vi "pressure system controller v14 motor.vi"() -> ()   [LabVIEW 2009]
uses:
  <vilib>/DAQmx/create/channels.llb/DAQmx Create Channel (DO-Digital Output).vi
  <vilib>/Instr/_visa.llb/VISA Configure Serial Port (Instr).vi
  <vilib>/DAQmx/write.llb/DAQmx Write (Digital 1D Bool 1Chan 1Samp).vi
  <instrlib>/Keithley 24XX/Public/Data/Read (Single Point).vi
  <vilib>/express/express signal manip/GetorSetDDTAttributes/Set DDT Attributes/Set DDT Properties.xnode
  <vilib>/express/express shared/transition.llb/Waveform Array To Dynamic.vi
  <vilib>/express/express signal manip/GetorSetDDTAttributes/Set DDT Attributes/SetT0.vi
  <vilib>/express/express shared/transition.llb/Dynamic To Waveform Array.vi
  <instrlib>/Keithley 24XX/Keithley 24XX.lvlib
  <instrlib>/Agilent E4980/Agilent E4980.lvlib
panel:
  in  "Pressure (mmHg)":i32
  out "error out":errorcluster
  in  "motor GO!":bool
  in  "stop":bool
  in  "MUX4: Keithley (-)":T1(radio)
  in  "MUX3: Keithley (+)":T1(radio)
  in  "MUX2: LCR (-)":T1(radio)
  in  "MUX1: LCR (+)":T1(radio)
  in  "Write to file":bool=TRUE caption="Enable"
  in  "Turn on (MAKE SURE TURN OFF)":bool=TRUE
  out "Impedance":dbl format="%^#_4e"
  out "Phase (deg)":dbl
  in  "Function (0: Cp-D)":u16(ring)=17 items=["Cp-D", "Cp-Q", "Cp-G", "Cp-Rp", "Cs-D", "Cs-Q", "Cs-Rs", "Lp-D", "Lp-Q", "Lp-G", "Lp-Rp", "Lp-Rdc", "Ls-D", "Ls-Q", "Ls-Rs", "Ls-Rdc", "R-X", "Z-thd", "Z-thr", "G-B", "Y-thd", "Y-thr", "Vdc-Idc"]
  in  "Signal Level (1.0 V)":dbl=1.0
  in  "Averaging Factor (1)":i32=1
  in  "Measurement Time (1: Medium)":u16(ring) items=["Short", "Medium", "Long"]
  in  "Signal Frequency":dbl=10000.0
  out "Resistance (Mohm)":dbl
  out "Current (uA)":sgl
  out "Voltage":sgl
  in  "Loop sample rate (samples per second)":dbl=5.0
  in  "Current duration (s)":dbl=2.0
  out "Time Counter":i32
  in  "Keithley Output (uA)":dbl=1.0
  in  "Compliance (V)":dbl=21.0
  in  "Inject Current":bool
  # "Switch"
  # "Keithley Settings"
  # "LCR Settings"
  # "1KHz for water"
  # "10KHz for PBS"
  # "1 uA minimum"
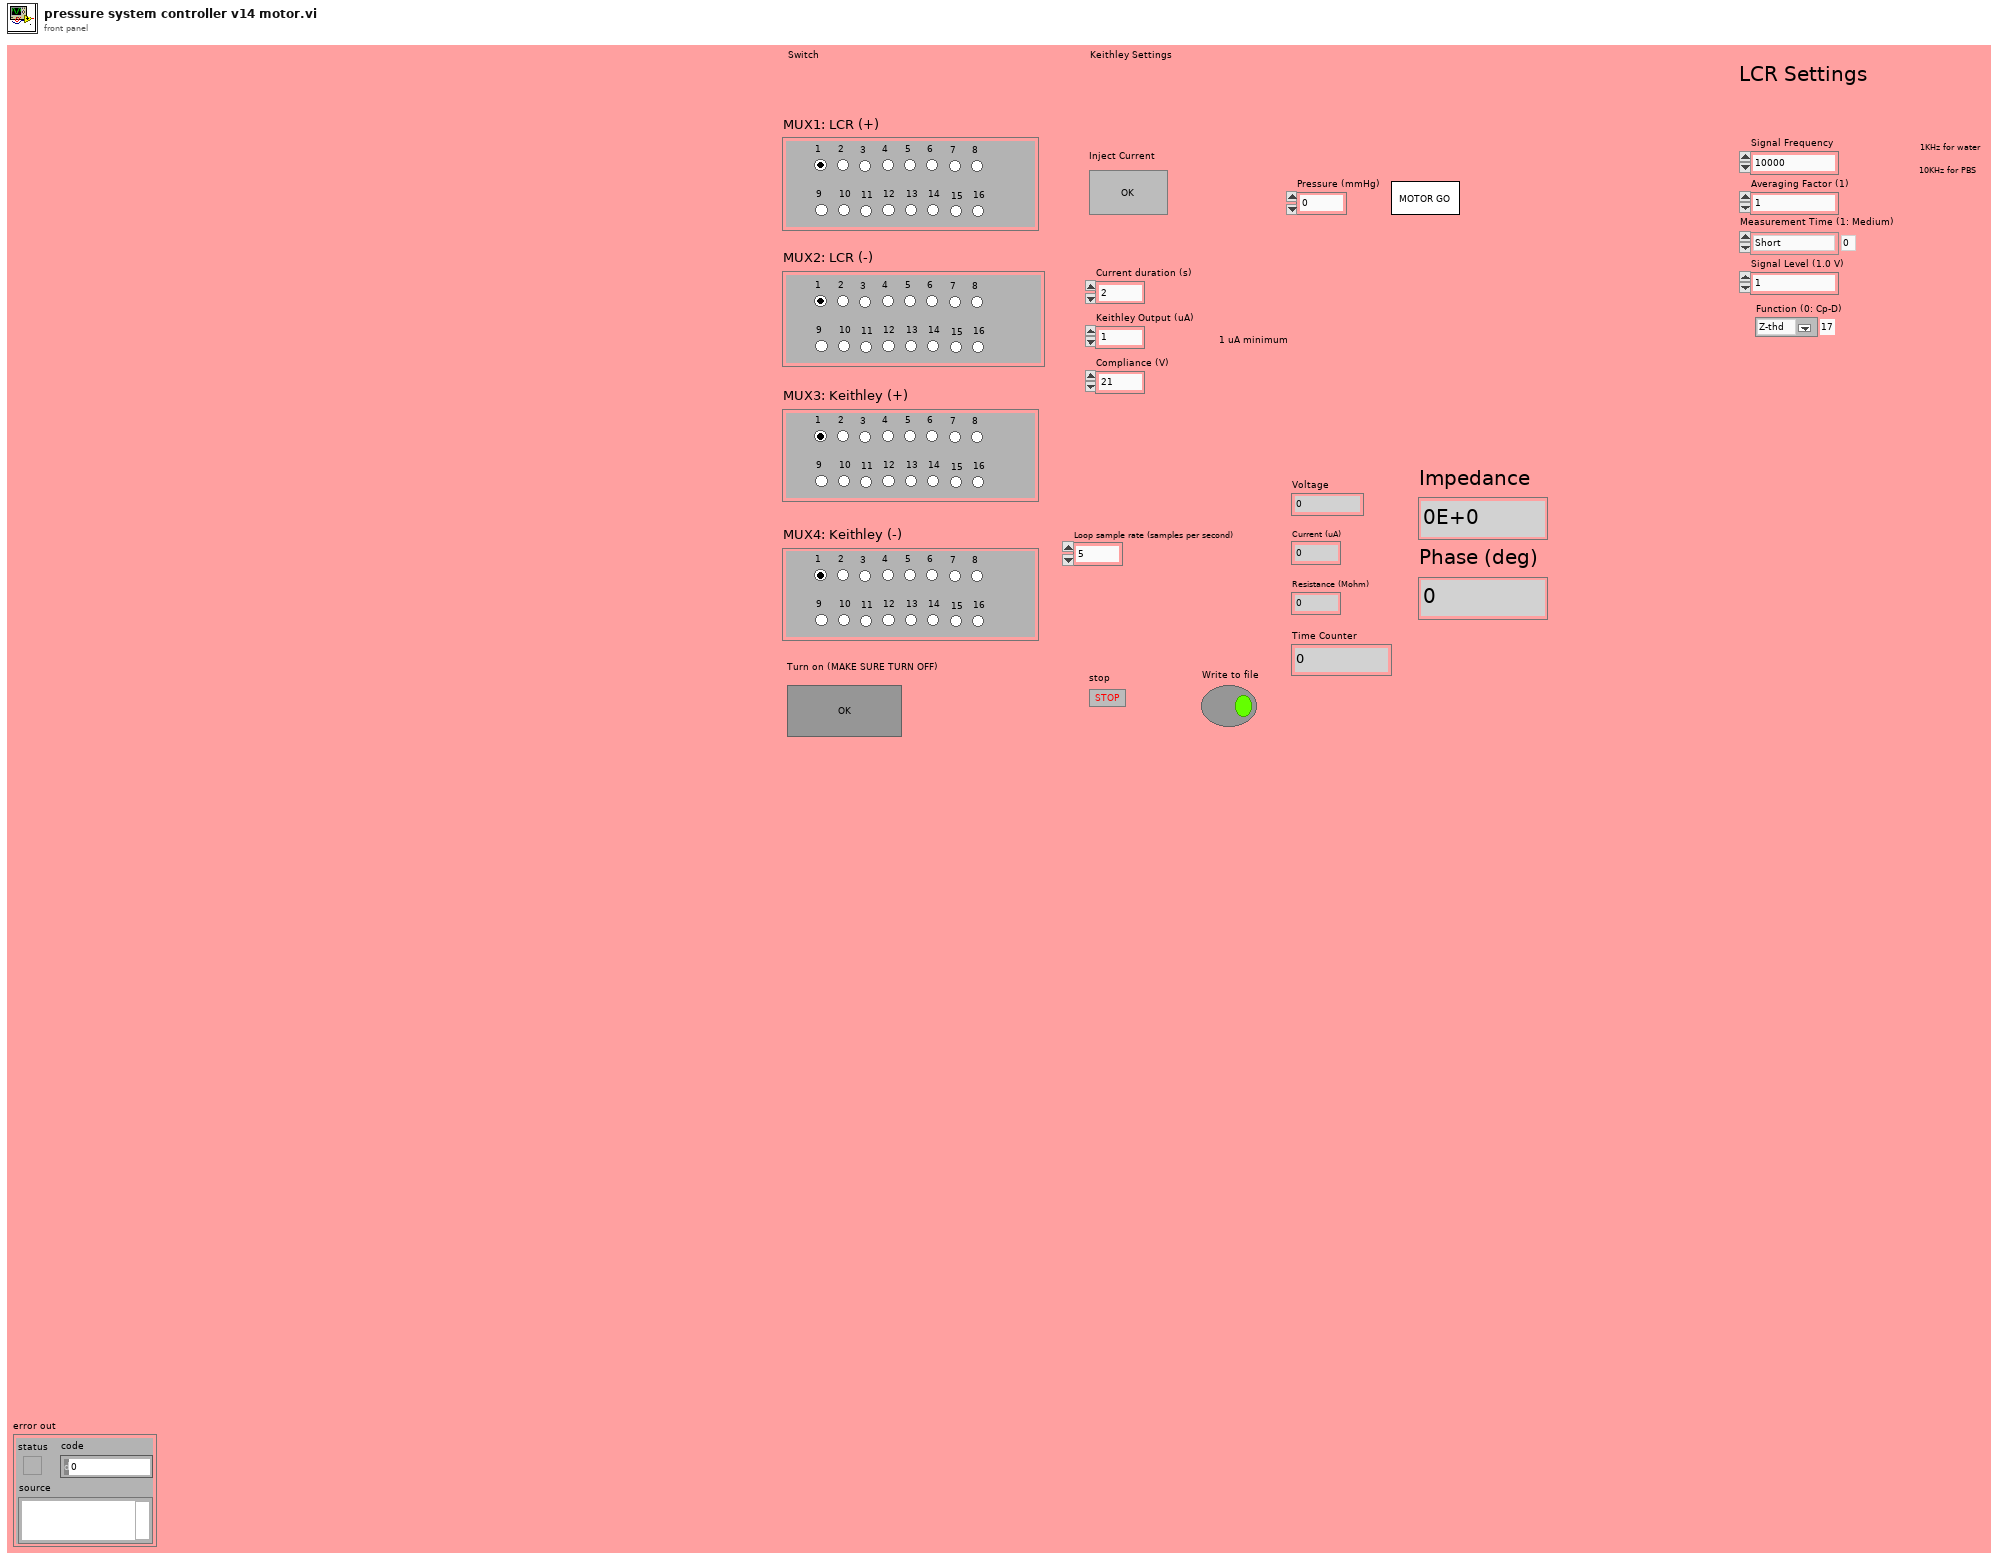
[diagram p1: front panel]
types:
  T1 = enum32{"1", "2", "3", "4", "5", "6", "7", "8", "9", "10", "11", "12", "13", "14", "15", "16"}
  T2 = cluster{"Primary Parameter":dbl, "Secondary Parameter":dbl}
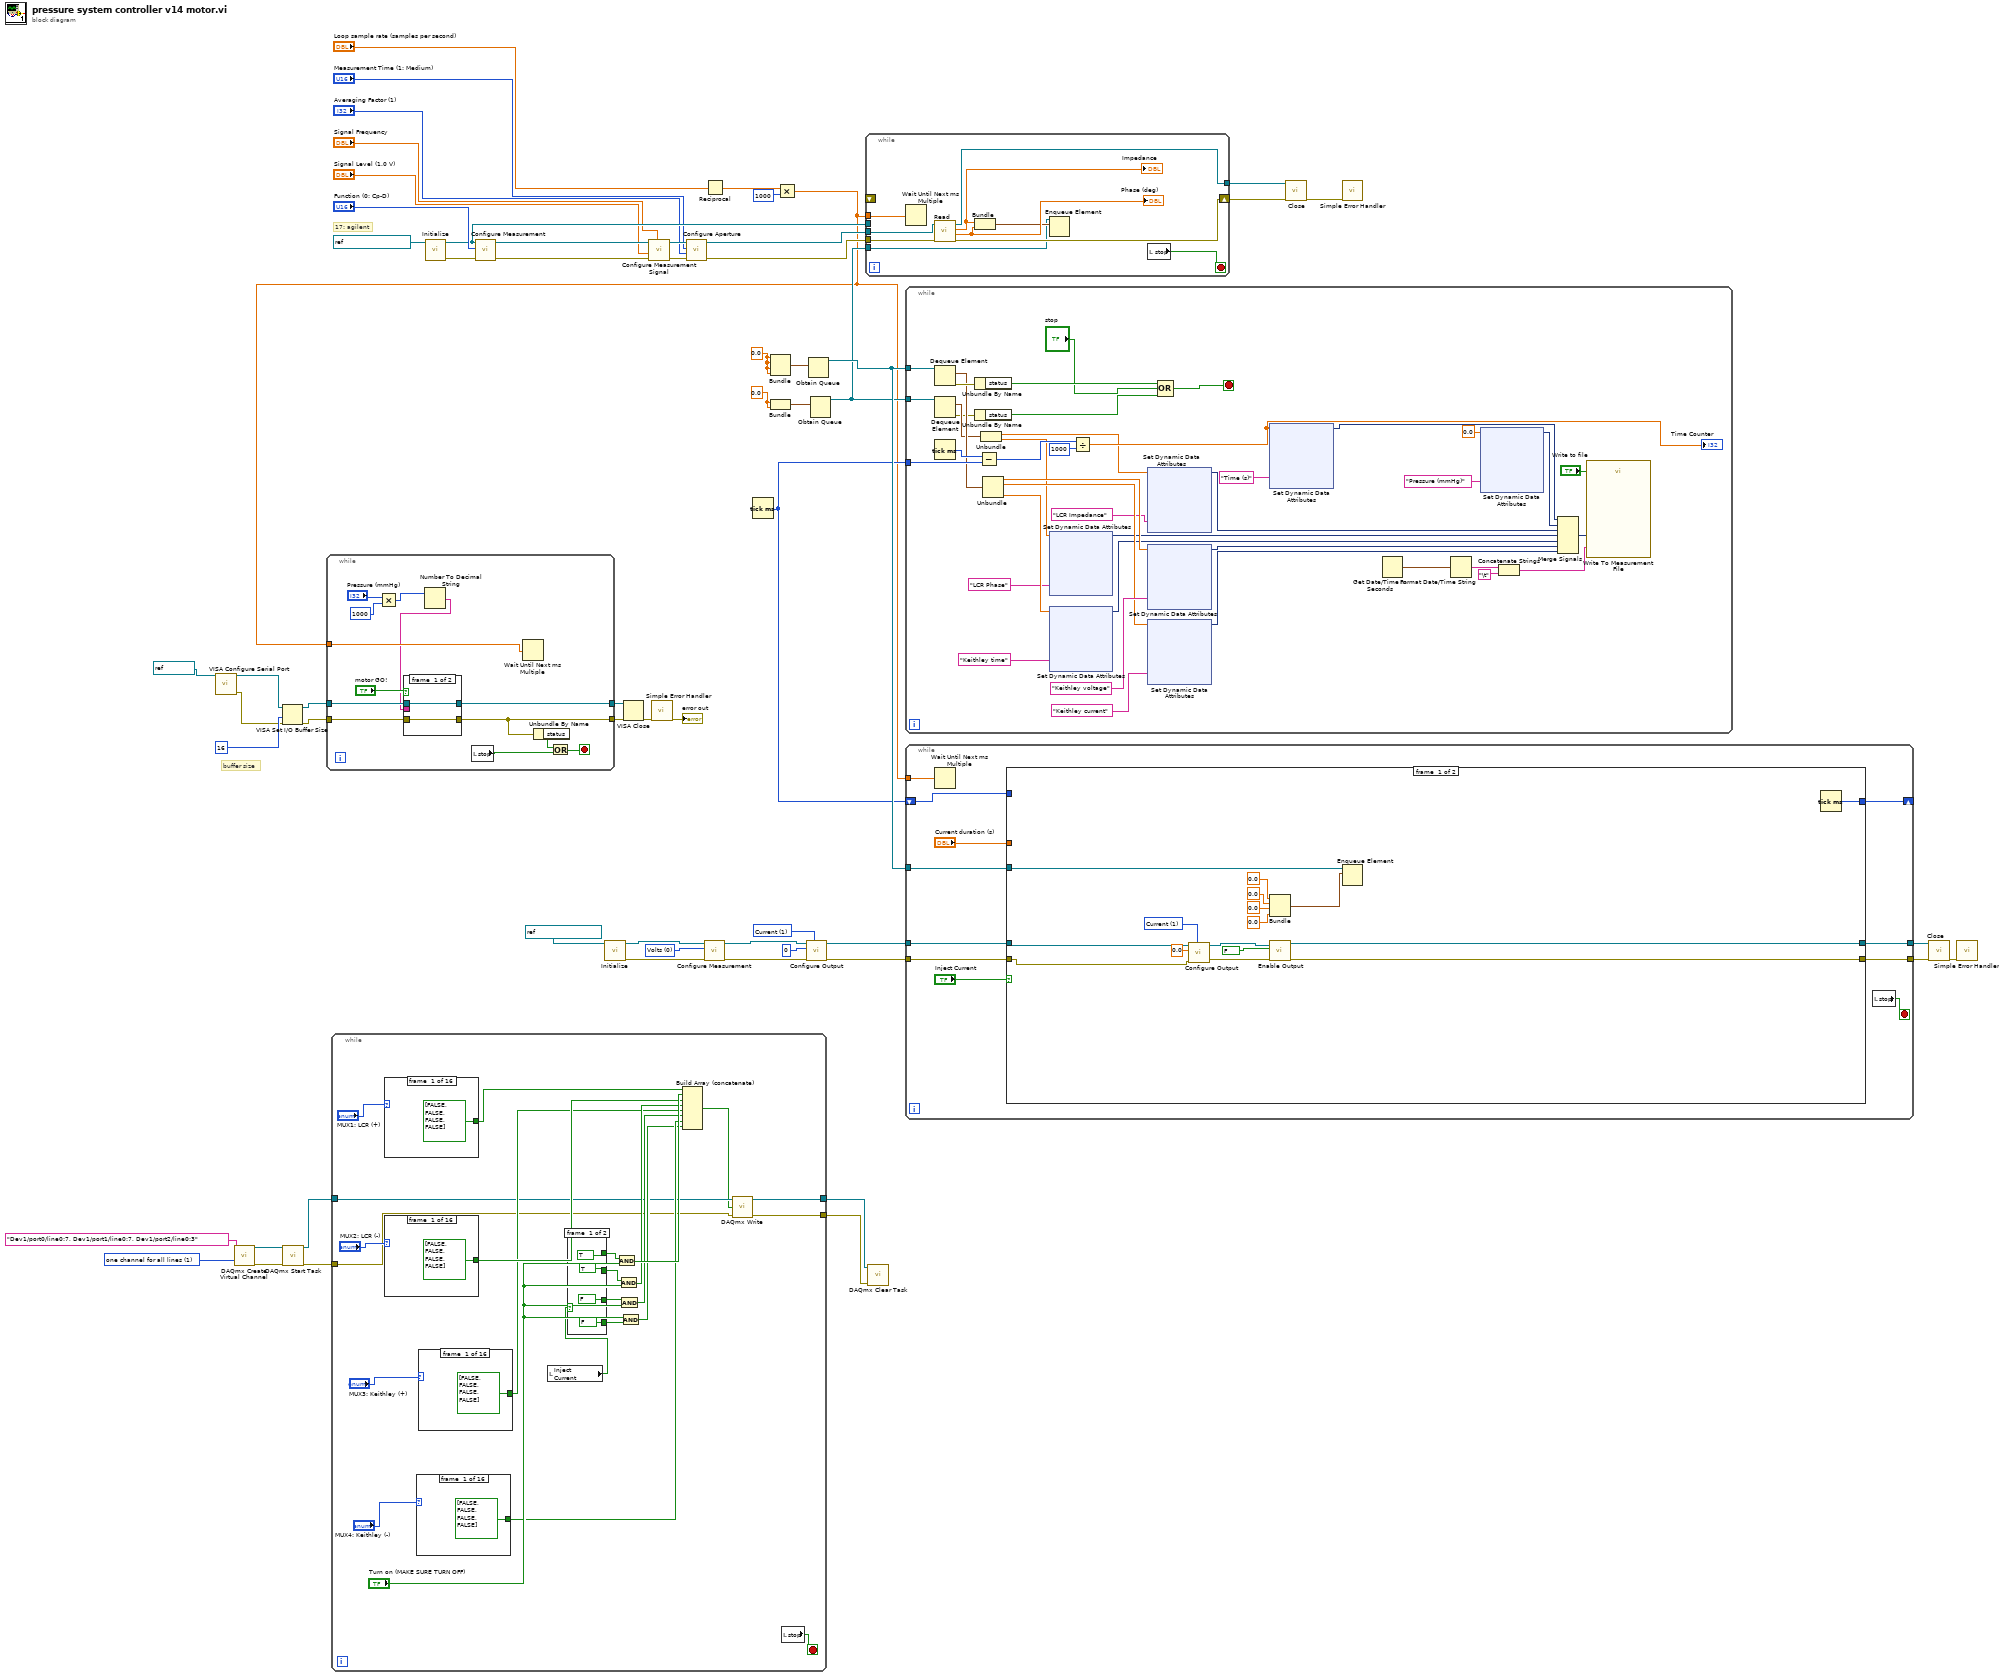
[diagram p0: block diagram]
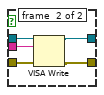
[diagram p2: hidden frame]
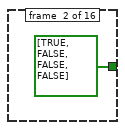
[diagram p3: hidden frame]
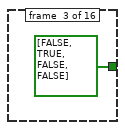
[diagram p4: hidden frame]
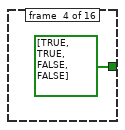
[diagram p5: hidden frame]
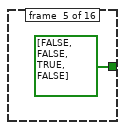
[diagram p6: hidden frame]
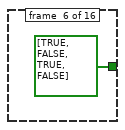
[diagram p7: hidden frame]
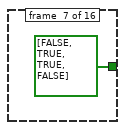
[diagram p8: hidden frame]
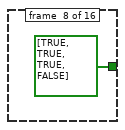
[diagram p9: hidden frame]
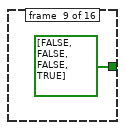
[diagram p10: hidden frame]
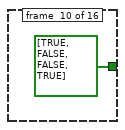
[diagram p11: hidden frame]
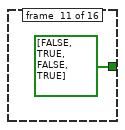
[diagram p12: hidden frame]
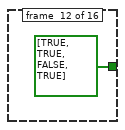
[diagram p13: hidden frame]
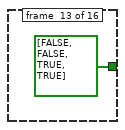
[diagram p14: hidden frame]
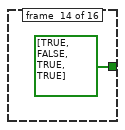
[diagram p15: hidden frame]
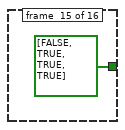
[diagram p16: hidden frame]
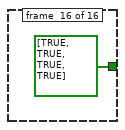
[diagram p17: hidden frame]
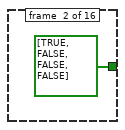
[diagram p18: hidden frame]
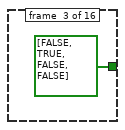
[diagram p19: hidden frame]
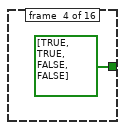
[diagram p20: hidden frame]
diagram:
  w20 = 1 items=["one channel for each line", "one channel for all lines"] ("line grouping")
  w53 = u16 1 items=["Voltage", "Current"] ("Source Mode  (0: Voltage)")
  w59 = u16 0 items=["Volts", "Current", "Resistance"] ("Keithley Measure")
  w39 = sgl 0.0 ("y")
  w47 = sgl 0.0 ("y")
  # "buffer size"
  # "17: agilent"
  n1 = call-poly "VISA Configure Serial Port"("VISA resource name"=refnum<visa-resource-name> "COM3") -> ("VISA resource name out"=w4:refnum<visa-resource-name>, "error out"=w3:errorcluster)  [unwired: 13 in]
  n2 = call-poly <vilib>:"DAQmx Create Virtual Channel.vi"("lines"=tag "Dev1/port0/line0:7, Dev1/port1/line0:7, Dev1/port2/line0:3", "line grouping"=w20) -> ("task out"=w18:refnum<k21>, "error out"=w19:errorcluster)  [unwired: 12 in]
  n3 = VISA Set I/O Buffer Size(VISA resource name=w4, size (4096)=u32 16 ("buffer size"), error in (no error)=w3) -> (VISA resource name out=w5:refnum<visa-resource-name>, error out=w6:errorcluster)  [unwired: 1 in]
  n4 = call <vilib>:"DAQmx Start Task.vi"("task/channels in"=w18, "error in"=w19) -> ("task out"=w16:refnum<k21>, "error out"=w14:errorcluster)  [unwired: 12 in]
  n5 = while {
    tunnel: w16 -> [w65]
    tunnel: [w64] -> w15
    tunnel: w14 -> [w63]
    tunnel: [w62] -> w13
    stop <- w82 stop-if-true
    n6 = case shown="\"1\", Default" "MUX1: LCR (+)" {
      tunnel: [bool[] [FALSE, FALSE, FALSE, FALSE] bool[] [TRUE, FALSE, FALSE, FALSE] bool[] [FALSE, TRUE, FALSE, FALSE] bool[] [TRUE, TRUE, FALSE, FALSE] bool[] [FALSE, FALSE, TRUE, FALSE] bool[] [TRUE, FALSE, TRUE, FALSE] bool[] [FALSE, TRUE, TRUE, FALSE] bool[] [TRUE, TRUE, TRUE, FALSE] bool[] [FALSE, FALSE, FALSE, TRUE] bool[] [TRUE, FALSE, FALSE, TRUE] bool[] [FALSE, TRUE, FALSE, TRUE] bool[] [TRUE, TRUE, FALSE, TRUE] bool[] [FALSE, FALSE, TRUE, TRUE] bool[] [TRUE, FALSE, TRUE, TRUE] bool[] [FALSE, TRUE, TRUE, TRUE] bool[] [TRUE, TRUE, TRUE, TRUE]] -> w73
      frame #0 {
      }
      frame #1 {
      }
      frame #2 {
      }
      frame #3 {
      }
      frame #4 {
      }
      frame #5 {
      }
      frame #6 {
      }
      frame #7 {
      }
      frame #8 {
      }
      frame #9 {
      }
      frame #10 {
      }
      frame #11 {
      }
      frame #12 {
      }
      frame #13 {
      }
      frame #14 {
      }
      frame #15 {
      }
    }
    n7 = case shown="\"1\", Default" "MUX2: LCR (-)" {
      tunnel: [bool[] [FALSE, FALSE, FALSE, FALSE] bool[] [TRUE, FALSE, FALSE, FALSE] bool[] [FALSE, TRUE, FALSE, FALSE] bool[] [TRUE, TRUE, FALSE, FALSE] bool[] [FALSE, FALSE, TRUE, FALSE] bool[] [TRUE, FALSE, TRUE, FALSE] bool[] [FALSE, TRUE, TRUE, FALSE] bool[] [TRUE, TRUE, TRUE, FALSE] bool[] [FALSE, FALSE, FALSE, TRUE] bool[] [TRUE, FALSE, FALSE, TRUE] bool[] [FALSE, TRUE, FALSE, TRUE] bool[] [TRUE, TRUE, FALSE, TRUE] bool[] [FALSE, FALSE, TRUE, TRUE] bool[] [TRUE, FALSE, TRUE, TRUE] bool[] [FALSE, TRUE, TRUE, TRUE] bool[] [TRUE, TRUE, TRUE, TRUE]] -> w71
      frame #0 {
      }
      frame #1 {
      }
      frame #2 {
      }
      frame #3 {
      }
      frame #4 {
      }
      frame #5 {
      }
      frame #6 {
      }
      frame #7 {
      }
      frame #8 {
      }
      frame #9 {
      }
      frame #10 {
      }
      frame #11 {
      }
      frame #12 {
      }
      frame #13 {
      }
      frame #14 {
      }
      frame #15 {
      }
    }
    n8 = case shown="\"2\"" "MUX4: Keithley (-)" {
      tunnel: [bool[] [FALSE, FALSE, FALSE, FALSE] bool[] [TRUE, FALSE, FALSE, FALSE] bool[] [FALSE, TRUE, FALSE, FALSE] bool[] [TRUE, TRUE, FALSE, FALSE] bool[] [FALSE, FALSE, TRUE, FALSE] bool[] [TRUE, FALSE, TRUE, FALSE] bool[] [FALSE, TRUE, TRUE, FALSE] bool[] [TRUE, TRUE, TRUE, FALSE] bool[] [FALSE, FALSE, FALSE, TRUE] bool[] [TRUE, FALSE, FALSE, TRUE] bool[] [FALSE, TRUE, FALSE, TRUE] bool[] [TRUE, TRUE, FALSE, TRUE] bool[] [FALSE, FALSE, TRUE, TRUE] bool[] [TRUE, FALSE, TRUE, TRUE] bool[] [FALSE, TRUE, TRUE, TRUE] bool[] [TRUE, TRUE, TRUE, TRUE]] -> w67
      frame #0 {
      }
      frame #1 {
      }
      frame #2 {
      }
      frame #3 {
      }
      frame #4 {
      }
      frame #5 {
      }
      frame #6 {
      }
      frame #7 {
      }
      frame #8 {
      }
      frame #9 {
      }
      frame #10 {
      }
      frame #11 {
      }
      frame #12 {
      }
      frame #13 {
      }
      frame #14 {
      }
      frame #15 {
      }
    }
    n9 = case shown="\"1\", Default" "MUX3: Keithley (+)" {
      tunnel: [bool[] [FALSE, FALSE, FALSE, FALSE] bool[] [TRUE, FALSE, FALSE, FALSE] bool[] [FALSE, TRUE, FALSE, FALSE] bool[] [TRUE, TRUE, FALSE, FALSE] bool[] [FALSE, FALSE, TRUE, FALSE] bool[] [TRUE, FALSE, TRUE, FALSE] bool[] [FALSE, TRUE, TRUE, FALSE] bool[] [TRUE, TRUE, TRUE, FALSE] bool[] [FALSE, FALSE, FALSE, TRUE] bool[] [TRUE, FALSE, FALSE, TRUE] bool[] [FALSE, TRUE, FALSE, TRUE] bool[] [TRUE, TRUE, FALSE, TRUE] bool[] [FALSE, FALSE, TRUE, TRUE] bool[] [TRUE, FALSE, TRUE, TRUE] bool[] [FALSE, TRUE, TRUE, TRUE] bool[] [TRUE, TRUE, TRUE, TRUE]] -> w69
      frame #0 {
      }
      frame #1 {
      }
      frame #2 {
      }
      frame #3 {
      }
      frame #4 {
      }
      frame #5 {
      }
      frame #6 {
      }
      frame #7 {
      }
      frame #8 {
      }
      frame #9 {
      }
      frame #10 {
      }
      frame #11 {
      }
      frame #12 {
      }
      frame #13 {
      }
      frame #14 {
      }
      frame #15 {
      }
    }
    n10 = local read "Inject Current"() -> (w60:bool)
    n11 = case shown="False" w60 {
      tunnel: [TRUE FALSE] -> w77
      tunnel: [TRUE FALSE] -> w76
      tunnel: [FALSE TRUE] -> w75
      tunnel: [FALSE TRUE] -> w74
      frame #0 {
      }
      frame #1 {
      }
    }
    n12 = And(x=w77, y="Turn on (MAKE SURE TURN OFF)") -> (x .and. y?=w72:bool)
    n13 = And(x=w76, y="Turn on (MAKE SURE TURN OFF)") -> (x .and. y?=w70:bool)
    n14 = And(x=w75, y="Turn on (MAKE SURE TURN OFF)") -> (x .and. y?=w68:bool)
    n15 = And(x="Turn on (MAKE SURE TURN OFF)", y=w74) -> (x .and. y?=w66:bool)
    n16 = Build Array (concatenate)(w73, w72, w71, w70, w69, w68, w67, w66) -> (w61:bool[])
    n17 = call-poly <vilib>:"DAQmx Write.vi"("task/channels in"=w65, "data"=w61, "error in"=w63) -> ("task out"=w64:refnum<k21>, "error out"=w62:errorcluster)  [unwired: 10 in, 1 out]
    n18 = local read "stop"() -> (w82:bool)
  }
  n19 = call <instrlib>:"Initialize.vi"("VISA resource name"=refnum<visa-resource-name> "GPIB0::17::INSTR") -> ("error out"=w33:errorcluster, "VISA resource name out"=w32:refnum<visa-resource-name>)  [unwired: 9 in]
  n20 = call <instrlib>:"Configure Measurement.vi"("error in (no error)"=w33, "Function (0: Cp-D)"="Function (0: Cp-D)", "VISA resource name"=w32) -> ("error out"=w31:errorcluster, "VISA resource name out"=w30:refnum<visa-resource-name>)  [unwired: 7 in]
  n21 = call <instrlib>:"Initialize.vi"("VISA resource name"=refnum<visa-resource-name> "GPIB0::24::INSTR") -> ("error out"=w57:errorcluster, "VISA resource name out"=w58:refnum<visa-resource-name>)  [unwired: 9 in]
  n22 = call <instrlib>:"Configure Measurement Signal.vi"("Signal Frequency (1000 Hz)"="Signal Frequency", "error in (no error)"=w31, "Signal Level (1.0 V)"="Signal Level (1.0 V)", "VISA resource name"=w30) -> ("error out"=w27:errorcluster, "VISA resource name out"=w26:refnum<visa-resource-name>)  [unwired: 6 in]
  n23 = call <instrlib>:"Configure Aperture.vi"("error in (no error)"=w27, "Averaging Factor (1)"="Averaging Factor (1)", "Measurement Time (1: Medium)"="Measurement Time (1: Medium)", "VISA resource name"=w26) -> ("error out"=w23:errorcluster, "VISA resource name out"=w22:refnum<visa-resource-name>)  [unwired: 6 in]
  n24 = call <instrlib>:"Configure Measurement.vi"("error in (no error)"=w57, "Function (0: Volts)"=w59, "VISA resource name"=w58) -> ("error out"=w55:errorcluster, "VISA resource name out"=w56:refnum<visa-resource-name>)  [unwired: 7 in]
  n25 = Reciprocal(x="Loop sample rate (samples per second)") -> (1/x=w44:dbl)
  n26 = Tick Count (ms)() -> (millisecond timer value=w12:u32)
  n27 = Bundle("y"=w47, "y"=w47, "y"=w47, "y"=w47) -> (w46:cluster{"y":sgl, "y":sgl, "y":sgl, "y":sgl})  [unwired: 1 in]
  n28 = Bundle("y"=w39, "y"=w39) -> (w38:cluster{"y":sgl, "y":sgl})  [unwired: 1 in]
  n29 = Multiply(x=w44, y=1000) -> (x*y=w2:dbl)
  n30 = while {
    tunnel: w5 -> [w166]
    tunnel: w6 -> [w165]
    tunnel: [w163] -> w11
    tunnel: [w162] -> w10
    tunnel: w2 -> [w161]
    stop <- w167 stop-if-true
    n31 = Multiply(x="Pressure (mmHg)", y=i16 1000) -> (x*y=w157:i32)
    n32 = Number To Decimal String(number=w157) -> (decimal integer string=w159:string)  [unwired: 1 in]
    n33 = case shown="True" "motor GO!" {
      tunnel: w166 -> [w170 w175]
      tunnel: w165 -> [w169 w174]
      tunnel: [w170 w173] -> w163
      tunnel: [w169 w172] -> w162
      tunnel: w159 -> [_ w171]
      frame #0 {
      }
      frame #1 {
        n34 = VISA Write(VISA resource name=w175, write buffer=w171, error in (no error)=w174) -> (VISA resource name out=w173:refnum<visa-resource-name>, error out=w172:errorcluster)  [unwired: 1 out]
      }
    }
    n35 = local read "stop"() -> (w160:bool)
    n36 = Wait Until Next ms Multiple(millisecond multiple=w161) -> ()  [unwired: 1 out]
    n37 = Unbundle By Name(w162) -> ("status"=w168:bool)
    n38 = Or(x=w168, y=w160) -> (x .or. y?=w167:bool)
  }
  n39 = VISA Close(VISA resource name=w11, error in (no error)=w10) -> (error out=w9:errorcluster)
  n40 = call <vilib>:"Simple Error Handler.vi"("error in (no error)"=w9) -> ("error out"=→"error out":errorcluster)  [unwired: 4 in, 4 out]
  n41 = call <instrlib>:"Configure Output.vi"("Source Mode  (0: Voltage)"=w53, "error in (no error)"=w55, "Output Level (0)"=0, "VISA resource name"=w56) -> ("error out"=w51:errorcluster, "VISA resource name out"=w52:refnum<visa-resource-name>)  [unwired: 6 in]
  n42 = Obtain Queue(element data type=w46) -> (queue out=w50:refnum<queue>)  [unwired: 4 in, 2 out]
  n43 = Obtain Queue(element data type=w38) -> (queue out=w37:refnum<queue>)  [unwired: 4 in, 2 out]
  n44 = while {
    shift-right: [w185] -> w41
    shift-left: _ -> [_]
    tunnel: w32 -> [_]
    tunnel: [w184] -> w40
    tunnel: w2 -> [w183]
    tunnel: w37 -> [w179]
    tunnel: w23 -> [w177]
    tunnel: w22 -> [w176]
    stop <- w178 stop-if-true
    n45 = Wait Until Next ms Multiple(millisecond multiple=w183) -> ()  [unwired: 1 out]
    n46 = call <instrlib>:"Read.vi"("error in (no error)"=w177, "VISA resource name"=w176) -> ("error out"=w185:errorcluster, "Secondary Parameter"=w182:dbl, "Primary Parameter"=w181:dbl, "VISA resource name out"=w184:refnum<visa-resource-name>)  [unwired: 6 in]
    "Phase (deg)" <- w182
    "Impedance" <- w181
    n47 = Bundle("Primary Parameter"=w181, "Secondary Parameter"=w182) -> (w180:T2)  [unwired: 1 in]
    n48 = Enqueue Element(queue=w179, element=w180) -> ()  [unwired: 2 in, 3 out]
    n49 = local read "stop"() -> (w178:bool)
  }
  n50 = call <vilib>:"DAQmx Clear Task.vi"("task in"=w15, "error in"=w13) -> ()  [unwired: 13 in, 1 out]
  n51 = while {
    tunnel: w12 -> [w216]
    tunnel: w50 -> [w212]
    tunnel: w37 -> [w200]
    stop <- w210 stop-if-true
    n52 = Dequeue Element(queue=w212) -> (element=w209:cluster{"y":sgl, "y":sgl, "y":sgl, "y":sgl}, error out=w211:errorcluster)  [unwired: 2 in, 2 out]
    n53 = Dequeue Element(queue=w200) -> (element=w199:cluster{"y":sgl, "y":sgl}, error out=w196:errorcluster)  [unwired: 2 in, 2 out]
    n54 = Tick Count (ms)() -> (millisecond timer value=w219:u32)
    n55 = Unbundle By Name(w211) -> ("status"=w188:bool)
    n56 = Unbundle By Name(w196) -> ("status"=w195:bool)
    n57 = Subtract(x=w219, y=w216) -> (x-y=w217:u32)
    n58 = Unbundle(w199) -> ("y"=w197:sgl, "y"=w198:sgl)
    n59 = Unbundle(w209) -> ("y"=w204:sgl, "y"=w203:sgl, "y"=w205:sgl)  [unwired: 1 out]
    n60 = xnode "Set Dynamic Data Attributes"("Signal Name"="LCR Phase", "Signals In"=w198) -> ("Signals Out"=w193:dynamicdata)  [unwired: 2 in, 1 out]
    n61 = xnode "Set Dynamic Data Attributes"("Signal Name"="Keithley time", "Signals In"=w205) -> ("Signals Out"=w192:dynamicdata)  [unwired: 2 in, 1 out]
    n62 = Divide(x=w217, y=1000) -> (x/y=w214:dbl)
    "Time Counter" <- w214
    n63 = xnode "Set Dynamic Data Attributes"("Signal Name"="LCR Impedance", "Signals In"=w197) -> ("Signals Out"=w194:dynamicdata)  [unwired: 2 in, 1 out]
    n64 = xnode "Set Dynamic Data Attributes"("Signal Name"="Keithley voltage", "Signals In"=w204) -> ("Signals Out"=w191:dynamicdata)  [unwired: 2 in, 1 out]
    n65 = xnode "Set Dynamic Data Attributes"("Signal Name"="Keithley current", "Signals In"=w203) -> ("Signals Out"=w190:dynamicdata)  [unwired: 2 in, 1 out]
    n66 = Compound Arithmetic op=OR(w188, "stop", w195) -> (w210:bool)
    n67 = xnode "Set Dynamic Data Attributes"("Signal Name"="Time (s)", "Signals In"=w214) -> ("Signals Out"=w213:dynamicdata)  [unwired: 2 in, 1 out]
    n68 = Get Date/Time In Seconds() -> (seconds since 1Jan1904=w223:timestamp)
    n69 = Format Date/Time String(seconds (now)=w223) -> (date/time string=w224:string)  [unwired: 2 in]
    n70 = xnode "Set Dynamic Data Attributes"("Signal Name"="Pressure (mmHg)", "Signals In"=0.0) -> ("Signals Out"=w221:dynamicdata)  [unwired: 2 in, 1 out]
    n71 = Concatenate Strings(w224, "\t") -> (w222:string)
    n72 = Merge Signals(w213, w221, w194, w193, w192, w191, w190) -> (w220:dynamicdata)
    n73 = call "Write To Measurement File"("Signals"=w220, "Enable"="Write to file", "Comment"=w222) -> ()  [unwired: 14 in, 3 out]
  }
  n74 = while {
    tunnel: w52 -> [w335]
    tunnel: w51 -> [w334]
    tunnel: w50 -> [w331]
    tunnel: [w326] -> w49
    tunnel: [w325] -> w48
    shift-right: [w329] -> _
    shift-left: w12 -> [w328]
    tunnel: w2 -> [w327]
    stop <- w332 stop-if-true
    n75 = Wait Until Next ms Multiple(millisecond multiple=w327) -> ()  [unwired: 1 out]
    n76 = case shown="True" "Inject Current" {
      selector: "Inject Current" -> [_ w358]
      tunnel: w335 -> [w341 w382]
      tunnel: w334 -> [w340 w381]
      tunnel: w331 -> [w349 w374]
      tunnel: "Current duration (s)" -> [_ w372]
      tunnel: [w351 w366] -> w326
      tunnel: [w350 w365] -> w325
      tunnel: [w343 w363] -> w329
      tunnel: w328 -> [_ w363]
      frame #0 {
        w336 = u16 1 items=["Voltage", "Current"] ("Source Mode  (0: Voltage)")
        n77 = call <instrlib>:"Configure Output.vi"("Source Mode  (0: Voltage)"=w336, "error in (no error)"=w340, "Output Level (0)"=0.0, "VISA resource name"=w341) -> ("error out"=w338:errorcluster, "VISA resource name out"=w339:refnum<visa-resource-name>)  [unwired: 6 in]
        n78 = Bundle("y"=sgl 0.0, "y"=sgl 0.0, "y"=sgl 0.0, "y"=sgl 0.0) -> (w348:cluster{"y":sgl, "y":sgl, "y":sgl, "y":sgl})  [unwired: 1 in]
        n79 = call <instrlib>:"Enable Output.vi"("error in (no error)"=w338, "Enable Output (T: Enable)"=FALSE, "VISA resource name"=w339) -> ("error out"=w350:errorcluster, "VISA resource name out"=w351:refnum<visa-resource-name>)  [unwired: 7 in]
        n80 = Enqueue Element(queue=w349, element=w348) -> ()  [unwired: 2 in, 3 out]
        n81 = Tick Count (ms)() -> (millisecond timer value=w343:u32)
      }
      frame #1 {
        w355 = u16 1 items=["Voltage", "Current"] ("Source Mode  (0: Voltage)")
        n82 = Tick Count (ms)() -> (millisecond timer value=w364:u32)
        n83 = Subtract(x=w364, y=w363) -> (x-y=w359:u32)
        n84 = call <instrlib>:"Enable Output.vi"("error in (no error)"=w381, "Enable Output (T: Enable)"=w358, "VISA resource name"=w382) -> ("error out"=w356:errorcluster, "VISA resource name out"=w357:refnum<visa-resource-name>)  [unwired: 7 in]
        n85 = Divide(x=w359, y=1000) -> (x/y=w369:dbl)
        n86 = Multiply(x="Keithley Output (uA)", y=1e-06) -> (x*y=w360:dbl)
        n87 = Greater Or Equal?(x=w369, y=w372) -> (x >= y?=w370:bool)
        n88 = Not(x=w370) -> (.not. x?=w371:bool)
        n89 = local write "Inject Current"(w371) -> ()
        n90 = call <instrlib>:"Configure Output.vi"("Source Mode  (0: Voltage)"=w355, "error in (no error)"=w356, "Compliance  Level (0.1)"="Compliance (V)", "Output Level (0)"=w360, "VISA resource name"=w357) -> ("error out"=w352:errorcluster, "VISA resource name out"=w353:refnum<visa-resource-name>)  [unwired: 5 in]
        n91 = call-poly <instrlib>:"Read.vi"("VISA resource name"=w353, "error in (no error)"=w352) -> ("Voltage"=w368:sgl, "VISA resource name out"=w366:refnum<visa-resource-name>, "Current"=w380:sgl, "Resistance"=w378:sgl, "error out"=w365:errorcluster)  [unwired: 7 in, 2 out]
        "Voltage" <- w368
        n92 = Multiply(x=w378, y=1e-06) -> (x*y=w376:dbl)
        "Resistance (Mohm)" <- w376
        n93 = Multiply(x=w380, y=sgl 1000000.0) -> (x*y=w367:sgl)
        "Current (uA)" <- w367
        n94 = Bundle("Voltage"=w368, w367, w376, w369) -> (w375:cluster{"Voltage":sgl, sgl, dbl, dbl})  [unwired: 1 in]
        n95 = Enqueue Element(queue=w374, element=w375) -> ()  [unwired: 2 in, 3 out]
      }
    }
    n96 = local read "stop"() -> (w332:bool)
  }
  n97 = call <instrlib>:"Close.vi"("error in (no error)"=w41, "VISA resource name"=w40) -> ("error out"=w35:errorcluster)  [unwired: 9 in]
  n98 = call <vilib>:"Simple Error Handler.vi"("error in (no error)"=w35) -> ()  [unwired: 4 in, 5 out]
  n99 = call <instrlib>:"Close.vi"("error in (no error)"=w48, "VISA resource name"=w49) -> ("error out"=w36:errorcluster)  [unwired: 9 in]
  n100 = call <vilib>:"Simple Error Handler.vi"("error in (no error)"=w36) -> ()  [unwired: 4 in, 5 out]
